vi "Read Entries.vi"(8 "error in (no error)":errorcluster, 11 "HighscoreDialog in":refnum<class "HighscoreDialog.lvclass">) -> (0 "error out":errorcluster, 2 "Entries":T1[](array[typedef]), 3 "HighscoreDialog out":refnum<class "HighscoreDialog.lvclass">)   [LabVIEW 2019, in "RT_Game.lvlib" / "HighscoreDialog.lvclass"]
uses:
  HighscoreDialog.lvclass
  Highscore/HighscoreEntry.ctl
  HighscoreDialog.lvclass/HighscoreDialog.ctl
  Highscore/Highscore.lvclass
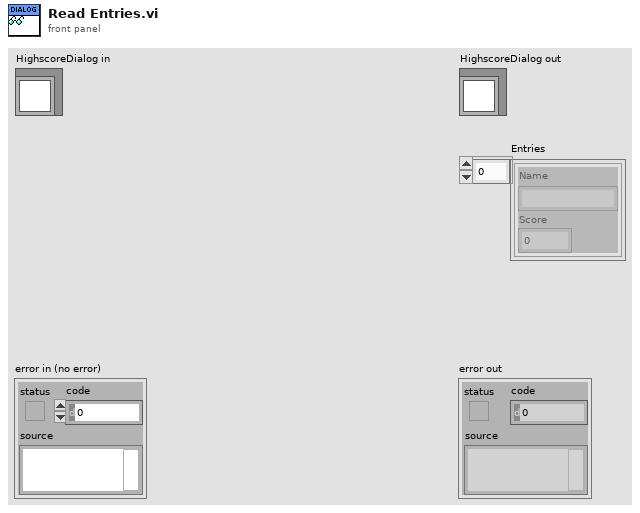
[diagram p1: front panel]
types:
  T1 = typedef "RT_Game.lvlib/Highscore.lvclass/HighscoreEntry.ctl" = cluster{"Name":string, "Score":dbl}
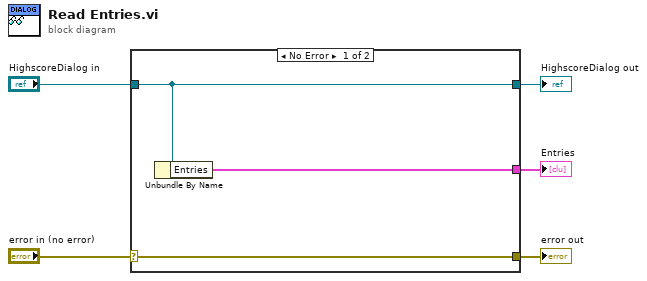
[diagram p0: block diagram]
diagram:
  n1 = case shown="No Error" "error in (no error)" {
    selector: "error in (no error)" -> [w8 w9]
    tunnel: [w8 w9] -> w4
    tunnel: [w7 w10] -> w2
    tunnel: "HighscoreDialog in" -> [w7 w10]
    tunnel: [w6 _] -> w1
    frame No Error {
      n2 = Unbundle By Name(w7) -> ("Entries"=w6:T1[])
    }
    frame Error {
    }
  }
  "error out" <- w4
  "HighscoreDialog out" <- w2
  "Entries" <- w1
